vi "start.vi"(8 "error in (no error)":errorcluster, 11 "SystemController in":refnum<class "SystemController.lvclass">) -> (0 "error out":errorcluster, 3 "SystemController out":refnum<class "SystemController.lvclass">)   [LabVIEW 2013, in "SystemController.lvclass"]
uses:
  SystemController.lvclass
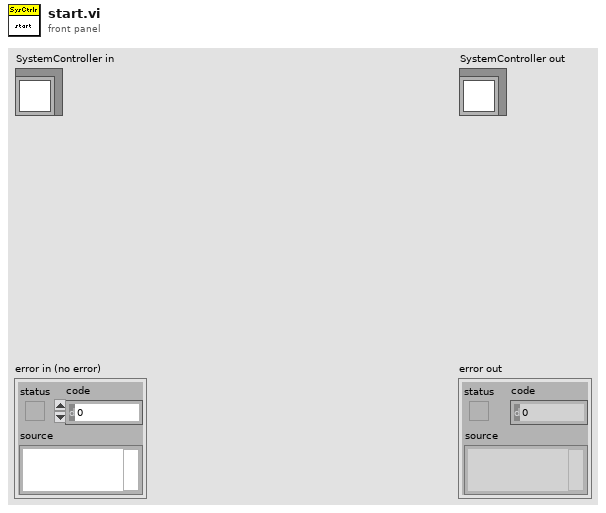
[diagram p1: front panel]
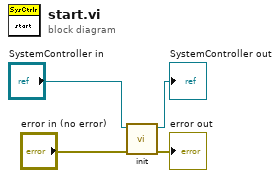
[diagram p0: block diagram]
diagram:
  n1 = call-dynamic "init.vi"("error in (no error)"="error in (no error)", "Compensator in"="SystemController in") -> ("error out"=→"error out":errorcluster, "Compensator out"=→"SystemController out":refnum<class "SystemController.lvclass">)  [unwired: 8 in]
